vi "Sort Cut-Outs.vi"(8 "error in (no error)":errorcluster, 11 "Exc Info in":T1[](array[typedef])) -> (0 "error out":errorcluster, 3 "Exc Info out":T1[](array[typedef]))   [LabVIEW 2024]
uses:
  Controls/Excluded Information.ctl
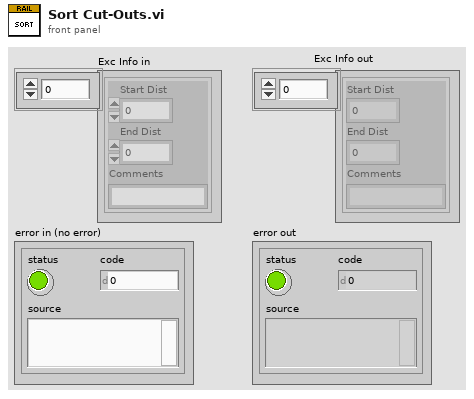
[diagram p1: front panel]
types:
  T1 = typedef "Excluded Information.ctl" = cluster{"Start Dist":dbl, "End Dist":dbl, "Comments":string}
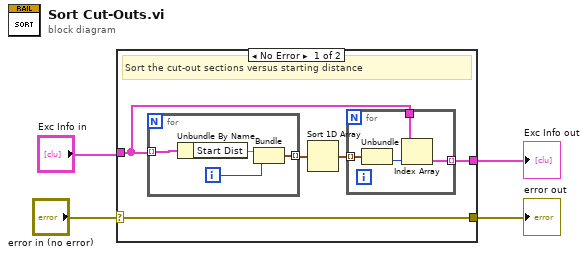
[diagram p0: block diagram]
diagram:
  n1 = case shown="No Error" "error in (no error)" {
    selector: "error in (no error)" -> [w5 w18]
    tunnel: "Exc Info in" -> [w7 w19]
    tunnel: [w6 w19] -> w2
    tunnel: [w5 w18] -> w4
    frame No Error {
      # "Sort the cut-out sections versus starting distance"
      n2 = for {
        tunnel: w7 -> [w15] mode=indexing
        tunnel: [w16] -> w8 mode=indexing
        i -> [w17]
        n3 = Unbundle By Name(w15) -> ("Start Dist"=w14:dbl)
        n4 = Bundle("Start Dist"=w14, w17) -> (w16:cluster{"Start Dist":dbl, i32})  [unwired: 1 in]
      }
      n5 = Sort 1D Array(array=w8) -> (sorted array=w9:cluster{"Start Dist":dbl, i32}[])
      n6 = for {
        tunnel: w9 -> [w13] mode=indexing
        tunnel: [w11] -> w6 mode=indexing
        tunnel: w7 -> [w12]
        n7 = Unbundle(w13) -> (w10:i32)  [unwired: 1 out]
        n8 = Index Array(array=w12, index=w10) -> (element=w11:T1)
      }
    }
    frame Error {
    }
  }
  "error out" <- w4
  "Exc Info out" <- w2
